vi "Drive Controller.vi"(8 "error out":errorcluster) -> ()   [LabVIEW 2016, in "Drive System.lvlib"]
uses:
  Drive System.lvlib
  Private/DriveCmdList.ctl
  Private/DriveCmd.ctl
  Private/DriveMainType.ctl
  <vilib>/Rock Robotics/WPI/RobotDrive/WPI_RobotDriveDevRef.ctl
  <vilib>/Rock Robotics/WPI/MotorControl/WPI_MotorControlDeviceRef.ctl
  <vilib>/Rock Robotics/WPI/MotorControl/WPI_MotorControlType.ctl
  <vilib>/Rock Robotics/SystemInterfaces/DIO/FPGA_DIOPWMChannel.ctl
  <vilib>/Rock Robotics/WPI/PWM/WPI_PWMDeadband.ctl
  <vilib>/Rock Robotics/WPI/Encoder/WPI_EncoderDevRef.ctl
  <vilib>/Rock Robotics/SystemInterfaces/Encoder/FPGA_EncoderIdx.ctl
  <vilib>/Rock Robotics/SystemInterfaces/Counter/FPGA_CounterCtrSystemIndex.ctl
  <vilib>/Rock Robotics/WPI/Encoder/WPI_EncoderType.ctl
  <vilib>/Rock Robotics/WPI/Gyro/WPI_GyroDevRef.ctl
  <vilib>/Rock Robotics/SystemInterfaces/AI/FPGA_AIChannel.ctl
  <vilib>/Rock Robotics/SystemInterfaces/spilib/spi_bus.ctl
  Private/Varient Cmd Types/Lock Command.ctl
  <vilib>/Rock Robotics/WPI/Solenoid/WPI_SolenoidDevRef.ctl
  <vilib>/Rock Robotics/WPI/Solenoid/WPI_SolenoidChannel.ctl
  Private/Varient Cmd Types/Drive Tank.ctl
  Private/Varient Cmd Types/Drive Arcade.ctl
  Private/Varient Cmd Types/Drive Time.ctl
  Private/Varient Cmd Types/Follow Path.ctl
  Pathfinder/VIs/Segment.ctl
  Private/Raw Data.vi
  <vilib>/Rock Robotics/WPI/Utilities/WPI_GetSetVariantRefNum.vi
  <vilib>/Rock Robotics/Network Tables/NT Write Numeric Array.vi
  <vilib>/Rock Robotics/Network Tables/NT Write String.vi
  Pathfinder/Pathfinder.lvlib
  Private/Drive Refs/Drive Ref Type.ctl
panel:
  out "Locking VI":string
  out "Is Locked?":bool
  out "Active Command:":T1
  out "Visualize":T2(graph)
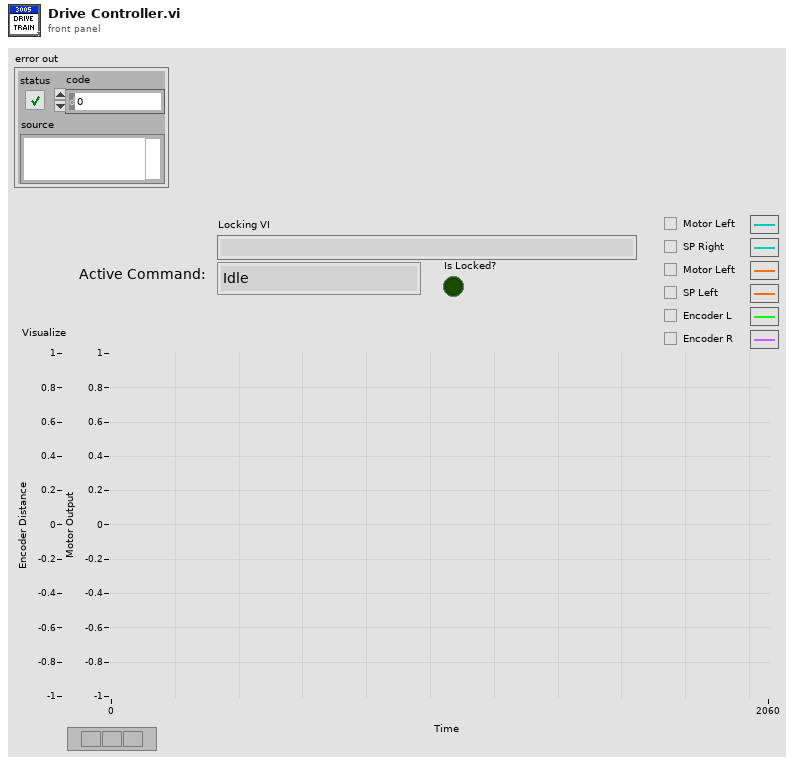
[diagram p1: front panel]
types:
  T1 = typedef "Drive System.lvlib/DriveCmdList.ctl" = enum16{"Idle", "Cleanup", "Drive For Time", "Follow Path Speed Control", "Follow Path", "Drive Tank", "Drive Straight PID", "Drive Angle Mag", "Drive Arcade", "Drive Ref", "Unlock", "Lock"}
  T2 = cluster{"Motor L":dbl, "SP L":dbl, "Motor R":dbl, "SP R":dbl, "Encoder L":dbl, "Encoder R":dbl}
  T3 = typedef "Drive System.lvlib/DriveMainType.ctl" = cluster{"queue":refnum<queue>, "Drivetrain":T4, "Encoder L":T9, "Encoder R":T9, "Gyro":T13, "Lock":T16, "Shifter":T17}
  T4 = typedef "WPI_RobotDriveDevRef.ctl" = cluster{"DevStatus":errorcluster, "Motors[]":T5[], "Square Inputs":bool, "Max Output":dbl}
  T5 = typedef "WPI_MotorControlDeviceRef.ctl" = cluster{"DeviceStatus":errorcluster, "Type":T6, "PWM":cluster{"PWM Channel":T7, "DeadBand":T8}, "CAN":cluster{"Device Number":u8, "SetOutput VI Ref":variant, "GetOutput VI Ref":variant, "Enable VI Ref":variant, "Disable VI Ref":variant, "Data":variant}, "Invert":bool}
  T6 = typedef "WPI_MotorControlType.ctl" = enum16{"PWM", "CAN"}
  T7 = typedef "FPGA_DIOPWMChannel.ctl" = enum8{"PWM 0", "PWM 1", "PWM 2", "PWM 3", "PWM 4", "PWM 5", "PWM 6", "PWM 7", "PWM 8", "PWM 9", "PWM MXP 0", "PWM MXP 1", "PWM MXP 2", "PWM MXP 3", "PWM MXP 4", "PWM MXP 5", "PWM MXP 6", "PWM MXP 7", "PWM MXP 8", "PWM MXP 9", "Invalid"}
  T8 = typedef "WPI_PWMDeadband.ctl" = cluster{"Name":string, "maxPositivePwm":i32, "minPositivePwm":i32, "centerPwm":i32, "maxNegativePwm":i32, "minNegativePwm":i32, "angularRange":u16}
  T9 = typedef "WPI_EncoderDevRef.ctl" = cluster{"DevStatus":errorcluster, "EncoderIndex":T10, "CounterIndex":T11, "DistancePerCount":dbl, "Decoding Type":T12}
  T10 = typedef "FPGA_EncoderIdx.ctl" = enum8{"Enc 0", "Enc 1", "Enc 2", "Enc 3", "Enc 4", "Enc 5", "Enc 6", "Enc 7", "Invalid"}
  T11 = typedef "FPGA_CounterCtrSystemIndex.ctl" = enum8{"Ctr 0", "Ctr 1", "Ctr 2", "Ctr 3", "Ctr 4", "Ctr 5", "Ctr 6", "Ctr 7", "Invalid"}
  T12 = typedef "WPI_EncoderType.ctl" = enum16{"1x", "2x", "4x"}
  T13 = typedef "WPI_GyroDevRef.ctl" = cluster{"DevStatus":errorcluster, "Analog Channel":T14, "Offset":dbl, "Gain (VoltsPerDegree/Second)":dbl, "Gyro Type":enum16{"Analog", "XRS450"}, "Handle":i32, "SPI Bus":T15, "Device Found":bool, "Sample Rate":dbl, "Calibrate On Open":bool}
  T14 = typedef "FPGA_AIChannel.ctl" = enum8{"AI 0", "AI 1", "AI 2", "AI 3", "AI MXP 0", "AI MXP 1", "AI MXP 2", "AI MXP 3", "Invalid"}
  T15 = typedef "spi_bus.ctl" = enum16{"SPI On-Board, CS0", "SPI On-Board, CS1", "SPI On-Board, CS2", "SPI On-Board, CS3", "SPI MXP", "Invalid"}
  T16 = typedef "Drive System.lvlib/Lock Command.ctl" = cluster{"notifier out":refnum<notifier>}
  T17 = typedef "WPI_SolenoidDevRef.ctl" = cluster{"DevStatus":errorcluster, "Pneumatics Control Module":u8, "Forward Solenoid Channel":T18, "Reverse Solenoid Channel":T18}
  T18 = typedef "WPI_SolenoidChannel.ctl" = enum8{"Solenoid 0", "Solenoid 1", "Solenoid 2", "Solenoid 3", "Solenoid 4", "Solenoid 5", "Solenoid 6", "Solenoid 7", "Invalid"}
  T19 = typedef "Drive System.lvlib/DriveCmd.ctl" = cluster{"cmd":T1, "data":variant, "Force? (F)":bool, "Lock":string}
  T20 = typedef "Drive System.lvlib/Drive Tank.ctl" = cluster{"Left":dbl, "Right":dbl}
  T21 = typedef "Drive System.lvlib/Drive Arcade.ctl" = cluster{"X Axis":dbl, "Y Axis":dbl}
  T22 = typedef "Drive System.lvlib/Drive Time.ctl" = cluster{"X Axis":dbl, "Y Axis":dbl, "Time (ms)":u32}
  T23 = typedef "Drive System.lvlib/Follow Path.ctl" = cluster{"Left":T24[], "Right":T24[]}
  T24 = typedef "Pathfinder.lvlib/Segment.ctl" = cluster{"dt":dbl, "x":dbl, "y":dbl, "position":dbl, "velocity":dbl, "acceleration":dbl, "jerk":dbl, "heading":dbl}
  T25 = typedef "Drive System.lvlib/Drive Ref Type.ctl" = refnum<vi>
  T26 = typedef "WPI_DriverStationRobotMode2.ctl" = enum16{"Autonomous Disabled", "Autonomous Enabled", "Teleop Disabled", "Teleop Enabled", "Disconnected", "Finish", "Test Disabled", "Test Enabled", "Emergency Stopped"}
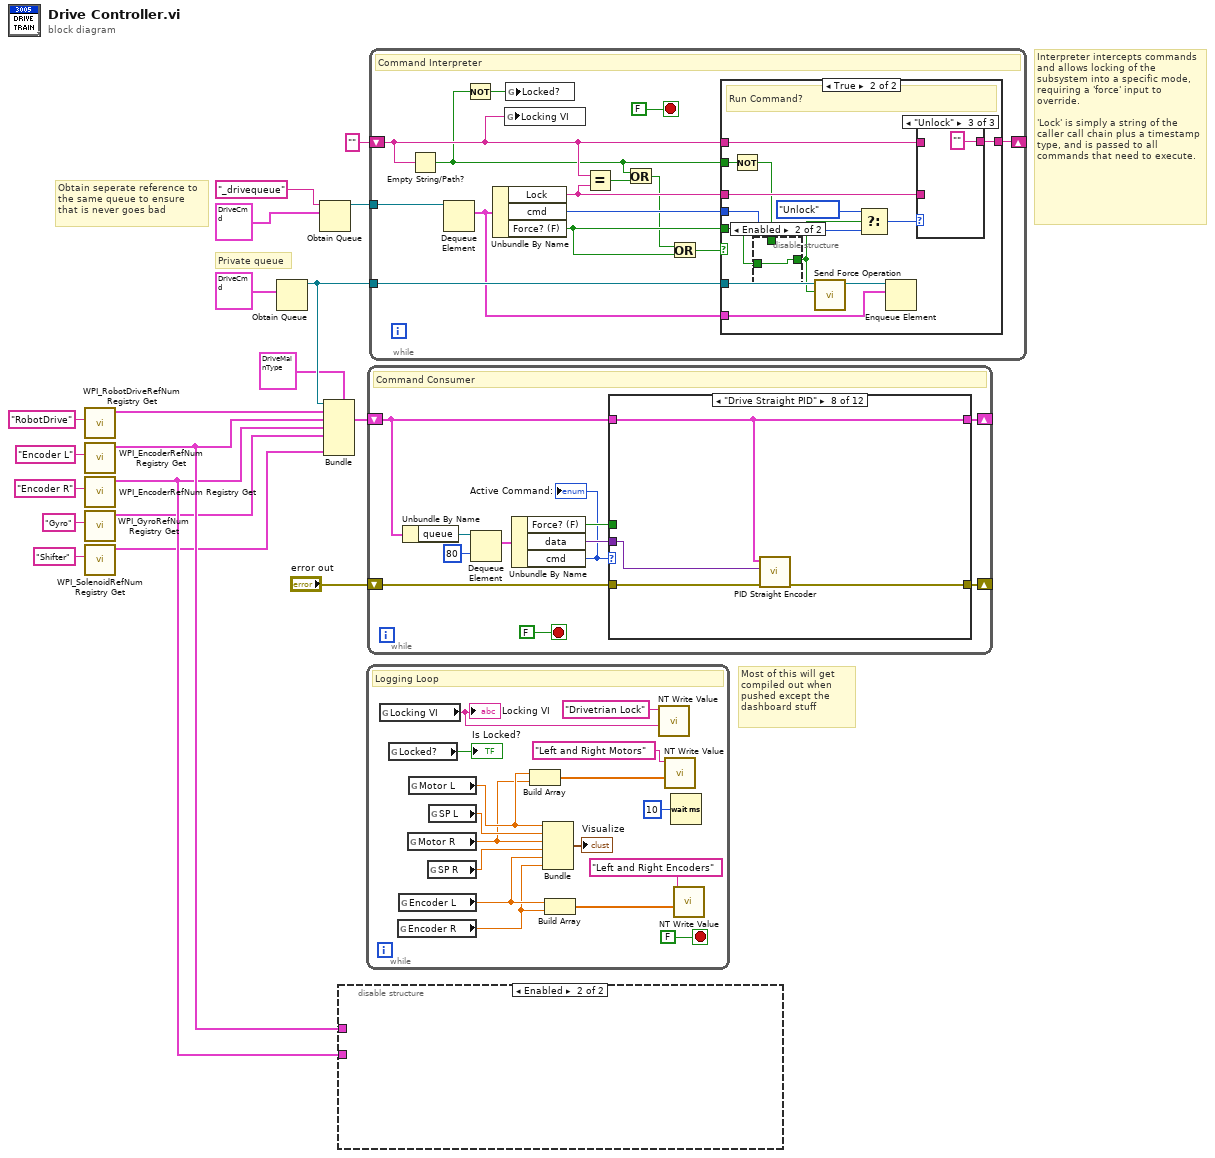
[diagram p0: block diagram]
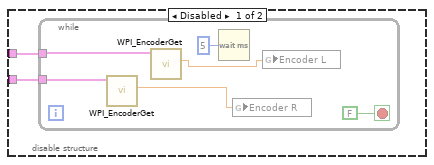
[diagram p2: hidden frame]
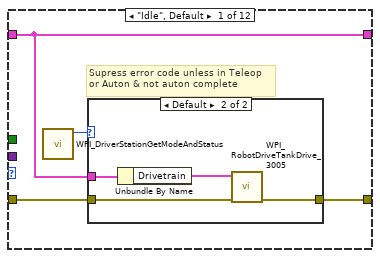
[diagram p3: hidden frame]
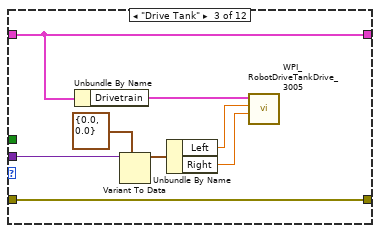
[diagram p6: hidden frame]
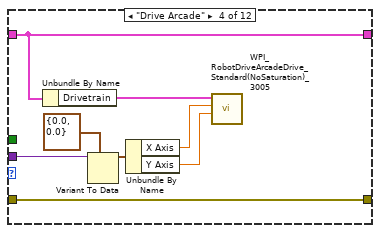
[diagram p7: hidden frame]
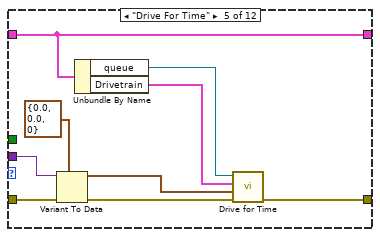
[diagram p8: hidden frame]
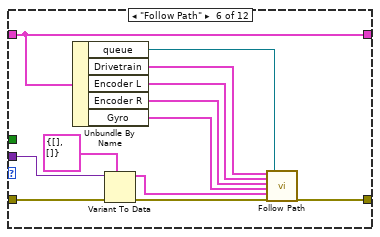
[diagram p9: hidden frame]
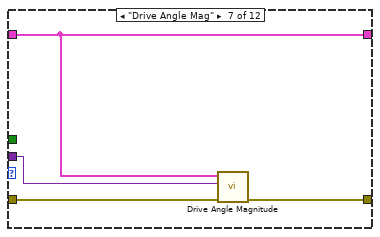
[diagram p10: hidden frame]
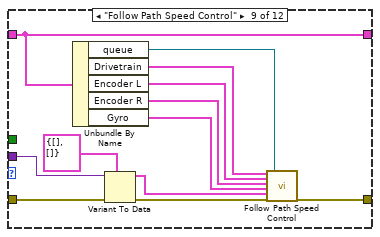
[diagram p11: hidden frame]
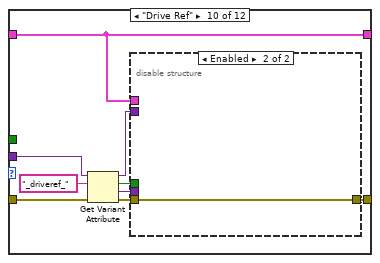
[diagram p12: hidden frame]
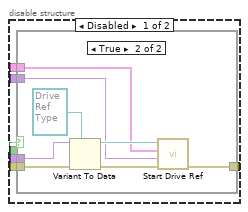
[diagram p13: hidden frame]
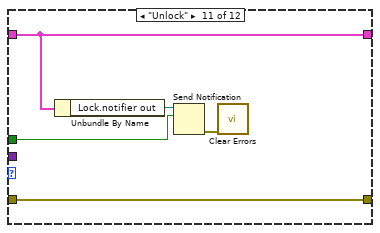
[diagram p15: hidden frame]
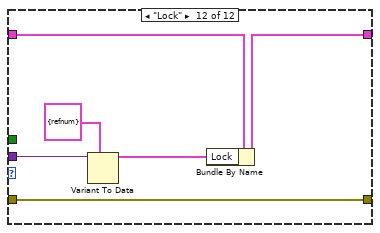
[diagram p16: hidden frame]
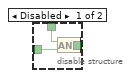
[diagram p18: hidden frame]
diagram:
  # "Most of this will get compiled out when pushed except the dashboard stuff"
  # "Interpreter intercepts commands and allows locking of the subsystem into a specific mode, requiring a 'force' input to override.\n\n'Lock' is simply a string of the caller call chain plus a timestamp type, and is passed to all commands that need to execute."
  # "Private queue"
  # "Obtain seperate reference to\nthe same queue to ensure\nthat is never goes bad"
  n1 = call <vilib>:"WPI_RobotDriveRefNum Registry Get.vi"("refnum name"="RobotDrive") -> ("RobotDriveDevRef"=w4:T4)  [unwired: 9 in, 1 out]
  n2 = call <vilib>:"WPI_EncoderRefNum Registry Get.vi"("refnum name"="Encoder L") -> ("EncoderDevRef"=w7:T9)  [unwired: 9 in, 1 out]
  n3 = call <vilib>:"WPI_EncoderRefNum Registry Get.vi"("refnum name"="Encoder R") -> ("EncoderDevRef"=w6:T9)  [unwired: 9 in, 1 out]
  n4 = call <vilib>:"WPI_GyroRefNum Registry Get.vi"("refnum name"="Gyro") -> ("GyroDevRef"=w5:T13)  [unwired: 9 in, 1 out]
  n5 = call <vilib>:"WPI_SolenoidRefNum Registry Get.vi"("refnum name"="Shifter") -> ("SolenoidDevRef"=w2:T17)  [unwired: 9 in, 1 out]
  n6 = Obtain Queue(element data type=T19 {"cmd"=enum."Cleanup", "data"=variant, "Force? (F)"=FALSE, "Lock"=""} ("Cluster")) -> (queue out=w19:refnum<queue>)  [unwired: 4 in, 2 out]
  n7 = Obtain Queue(name (unnamed)="_drivequeue", element data type=T19 {"cmd"=enum."Cleanup", "data"=variant, "Force? (F)"=FALSE, "Lock"=""}) -> (queue out=w14:refnum<queue>)  [unwired: 3 in, 2 out]
  n8 = Bundle(cluster=T3 {"queue"=refnum, "Drivetrain"={"DevStatus"={"status"=FALSE, "code"=0, "source"=""}, "Motors[]"=[], "Square Inputs"=FALSE, "Max Output"=0.0}, "Encoder L"={"DevStatus"={"status"=FALSE, "code"=0, "source"=""}, "EncoderIndex"=enum."Invalid", "CounterIndex"=enum."Invalid", "DistancePerCount"=1.0, "Decoding Type"=enum."4x"}, "Encoder R"={"DevStatus"={"status"=FALSE, "code"=0, "source"=""}, "EncoderIndex"=enum."Invalid", "CounterIndex"=enum."Invalid", "DistancePerCount"=1.0, "Decoding Type"=enum."4x"}, "Gyro"={"DevStatus"={"status"=FALSE, "code"=0, "source"=""}, "Analog Channel"=enum."Invalid", "Offset"=0.0, "Gain (VoltsPerDegree/Second)"=0.0, "Gyro Type"=enum."Analog", "Handle"=0, "SPI Bus"=enum."Invalid", "Device Found"=FALSE, "Sample Rate"=1.0, "Calibrate On Open"=FALSE}, "Lock"={"notifier out"=refnum}, "Shifter"={"DevStatus"={"status"=FALSE, "code"=0, "source"=""}, "Pneumatics Control Module"=0, "Forward Solenoid Channel"=enum."Invalid", "Reverse Solenoid Channel"=enum."Invalid"}}, "queue"=w19, "Drivetrain"=w4, "Encoder L"=w7, "Encoder R"=w6, "Gyro"=w5, "Shifter"=w2) -> (w18:T3)  [unwired: 1 in]
  n9 = disable-structure shown="Enabled" {
    disable-tunnel: w6 -> [w21 _]
    disable-tunnel: w7 -> [w20 _]
    frame Disabled {
      n10 = while {
        tunnel: w21 -> [w26]
        tunnel: w20 -> [w27]
        stop <- FALSE stop-if-true
        n11 = call <vilib>:"WPI_EncoderGet.vi"("EncoderDevRef"=w26) -> ("Distance"=w22:dbl)  [unwired: 5 in, 5 out]
        n12 = call <vilib>:"WPI_EncoderGet.vi"("EncoderDevRef"=w27) -> ("Distance"=w23:dbl)  [unwired: 5 in, 5 out]
        n13 = Wait (ms)(milliseconds to wait=u32 5) -> ()  [unwired: 1 out]
        n14 = global write "Raw Data.vi" "Encoder R"(w22) -> ()
        n15 = global write "Raw Data.vi" "Encoder L"(w23) -> ()
      }
    }
    frame Enabled {
    }
  }
  n16 = while {
    stop <- FALSE stop-if-true
    # "Logging Loop"
    n17 = global read "Raw Data.vi" "Locking VI"() -> (w28:string)
    "Locking VI" <- w28
    n18 = global read "Raw Data.vi" "Locked?"() -> (→"Is Locked?":bool)
    n19 = global read "Raw Data.vi" "Encoder R"() -> (w31:dbl)
    n20 = global read "Raw Data.vi" "Encoder L"() -> (w32:dbl)
    n21 = global read "Raw Data.vi" "Motor R"() -> (w39:dbl)
    n22 = global read "Raw Data.vi" "Motor L"() -> (w40:dbl)
    n23 = global read "Raw Data.vi" "SP R"() -> (w42:dbl)
    n24 = global read "Raw Data.vi" "SP L"() -> (w43:dbl)
    n25 = Build Array(w40, w39) -> (w38:dbl[])
    n26 = Bundle("Motor L"=w40, "SP L"=w43, "Motor R"=w39, "SP R"=w42, "Encoder L"=w32, "Encoder R"=w31) -> (→"Visualize":T2)  [unwired: 1 in]
    n27 = Build Array(w32, w31) -> (w33:dbl[])
    n28 = call-poly <vilib>:"NT Write Value.vi"("String"=w28, "Name"="Drivetrian Lock") -> ()  [unwired: 9 in, 1 out]
    n29 = call-poly <vilib>:"NT Write Value.vi"("Numeric Array"=w38, "Name"="Left and Right Motors") -> ()  [unwired: 9 in, 1 out]
    n30 = Wait (ms)(milliseconds to wait=u32 10) -> ()  [unwired: 1 out]
    n31 = call-poly <vilib>:"NT Write Value.vi"("Numeric Array"=w33, "Name"="Left and Right Encoders") -> ()  [unwired: 9 in, 1 out]
  }
  n32 = while {
    shift-right: [w50] -> _
    shift-left: w18 -> [w51]
    shift-right: [w48] -> _
    shift-left: "error out" -> [w47]
    stop <- FALSE stop-if-true
    # "Command Consumer"
    n33 = Unbundle By Name(w51) -> ("queue"=w52:refnum<queue>)
    n34 = Dequeue Element(queue=w52, timeout in ms (-1)=80) -> (element=w53:T19)  [unwired: 1 in, 3 out]
    n35 = Unbundle By Name(w53) -> ("Force? (F)"=w45:bool, "data"=w49:variant, "cmd"=w44:T1)
    "Active Command:" <- w44
    n36 = case shown="\"Drive Straight PID\"" w44 {
      tunnel: w51 -> [w56 w64 w73 w81 w84 w100 w106 w107 w120 w123 w151 w157]
      tunnel: [w56 w64 w73 w81 w84 w100 w106 w107 w120 w123 w151 w154] -> w50
      tunnel: w49 -> [_ _ w72 w80 w90 w102 w105 w108 w122 w130 _ w155]
      tunnel: [w57 w65 w68 w74 w86 w97 w103 w109 w117 w126 w152 w158] -> w48
      tunnel: w47 -> [w58 w65 w68 w74 w89 w101 w104 w110 w121 w131 w152 w158]
      tunnel: w45 -> [_ _ _ _ _ _ _ _ _ _ w148 _]
      frame "Idle", Default {
        # "Supress error code unless in Teleop\nor Auton & not auton complete"
        n37 = call <vilib>:"WPI_DriverStationGetModeAndStatus.vi"() -> ("Robot Mode"=w55:T26)  [unwired: 10 in, 1 out]
        n38 = case shown="Default" w55 {
          tunnel: w58 -> [w59 w62]
          tunnel: [w59 w60] -> w57
          tunnel: w56 -> [_ w63]
          frame "Teleop Enabled" {
          }
          frame Default {
            n39 = Unbundle By Name(w63) -> ("Drivetrain"=w61:T4)
            n40 = call "WPI_RobotDriveTankDrive_3005.vi"("error in (no error)"=w62, "RobotDriveDevRef"=w61) -> ("error out"=w60:errorcluster)  [unwired: 8 in, 1 out]
          }
        }
      }
      frame "Cleanup" {
      }
      frame "Drive Tank" {
        n41 = Unbundle By Name(w73) -> ("Drivetrain"=w70:T4)
        n42 = Variant To Data(type=T20 {"Left"=0.0, "Right"=0.0}, Variant=w72) -> (data=w69:T20)  [unwired: 1 in, 1 out]
        n43 = Unbundle By Name(w69) -> ("Left"=w67:dbl, "Right"=w66:dbl)
        n44 = call "WPI_RobotDriveTankDrive_3005.vi"("Right axis value"=w66, "Left axis value"=w67, "RobotDriveDevRef"=w70) -> ()  [unwired: 7 in, 2 out]
      }
      frame "Drive Arcade" {
        n45 = Unbundle By Name(w81) -> ("Drivetrain"=w77:T4)
        n46 = Variant To Data(type=T21 {"X Axis"=0.0, "Y Axis"=0.0}, Variant=w80) -> (data=w79:T21)  [unwired: 1 in, 1 out]
        n47 = Unbundle By Name(w79) -> ("X Axis"=w76:dbl, "Y Axis"=w75:dbl)
        n48 = call "WPI_RobotDriveArcadeDrive_Standard(NoSaturation)_3005.vi"("Y axis value"=w75, "X axis value"=w76, "RobotDriveDevRef"=w77) -> ()  [unwired: 7 in, 2 out]
      }
      frame "Drive For Time" {
        n49 = Variant To Data(error in=w89, type=T22 {"X Axis"=0.0, "Y Axis"=0.0, "Time (ms)"=0} ("Cluster"), Variant=w90) -> (data=w83:T22, error out=w87:errorcluster)
        n50 = Unbundle By Name(w84) -> ("queue"=w85:refnum<queue>, "Drivetrain"=w82:T4)
        n51 = call "Drive for Time.vi"("error in"=w87, "Cluster"=w83, "Drivetrain"=w82, "Queue in"=w85) -> ("error out"=w86:errorcluster)  [unwired: 7 in]
      }
      frame "Follow Path" {
        n52 = Unbundle By Name(w100) -> ("queue"=w94:refnum<queue>, "Drivetrain"=w93:T4, "Encoder L"=w92:T9, "Encoder R"=w91:T9, "Gyro"=w95:T13)
        n53 = Variant To Data(error in=w101, type=T23 {"Left"=[], "Right"=[]}, Variant=w102) -> (data=w96:T23, error out=w98:errorcluster)
        n54 = call "Follow Path.vi"("Drivetrain"=w93, "Encoder L"=w92, "Encoder R"=w91, "Gyro"=w95, "Trajectory"=w96, "error in"=w98, "Queue in"=w94) -> ("error out"=w97:errorcluster)  [unwired: 12 in]
      }
      frame "Drive Angle Mag" {
        n55 = call "Drive Angle Magnitude.vi"("error in"=w104, "data"=w105, "DriveRef"=w106) -> ("error out"=w103:errorcluster)  [unwired: 8 in]
      }
      frame "Drive Straight PID" {
        n56 = call "PID Straight Encoder.vi"("error in"=w110, "data"=w108, "Auton Ref"=w107) -> ("error out"=w109:errorcluster)  [unwired: 8 in]
      }
      frame "Follow Path Speed Control" {
        n57 = Unbundle By Name(w120) -> ("queue"=w114:refnum<queue>, "Drivetrain"=w113:T4, "Encoder L"=w112:T9, "Encoder R"=w111:T9, "Gyro"=w115:T13)
        n58 = Variant To Data(error in=w121, type=T23 {"Left"=[], "Right"=[]}, Variant=w122) -> (data=w116:T23, error out=w118:errorcluster)
        n59 = call "Follow Path Speed Control.vi"("Drivetrain"=w113, "Encoder L"=w112, "Encoder R"=w111, "Gyro"=w115, "Trajectory"=w116, "error in"=w118, "Queue in"=w114) -> ("error out"=w117:errorcluster)  [unwired: 12 in]
      }
      frame "Drive Ref" {
        n60 = Get Variant Attribute(Variant=w130, name="_driveref_", error in=w131) -> (duplicate Variant=w124:variant, found=w125:bool, value=w128:variant, error out=w127:errorcluster)  [unwired: 1 in]
        n61 = disable-structure shown="Enabled" {
          disable-tunnel: w128 -> [w137 _]
          disable-tunnel: w127 -> [w136 w147]
          disable-tunnel: [w135 w147] -> w126
          disable-tunnel: w125 -> [w134 _]
          disable-tunnel: w124 -> [w133 _]
          disable-tunnel: w123 -> [w132 _]
          frame Disabled {
            n62 = case shown="True" w134 {
              tunnel: w137 -> [_ w145]
              tunnel: w136 -> [w138 w144]
              tunnel: [w138 w140] -> w135
              tunnel: w133 -> [_ w141]
              tunnel: w132 -> [_ w142]
              frame False {
              }
              frame True {
                n63 = Variant To Data(error in=w144, type=T25 refnum ("Drive Ref"), Variant=w145) -> (data=w143:T25, error out=w139:errorcluster)
                n64 = call "Start Drive Ref.vi"("error in"=w139, "Variant"=w141, "cluster"=w142, "VI in"=w143) -> ("error out"=w140:errorcluster)  [unwired: 7 in]
              }
            }
          }
          frame Enabled {
          }
        }
      }
      frame "Unlock" {
        n65 = Unbundle By Name(w151) -> ("Lock.notifier out"=w150:refnum<notifier>)
        n66 = Send Notification(notification=w148, notifier=w150) -> (error out=w149:errorcluster)  [unwired: 1 in, 1 out]
        n67 = call <vilib>:"Clear Errors.vi"("error in (no error)"=w149) -> ()  [unwired: 5 in, 2 out]
      }
      frame "Lock" {
        n68 = Variant To Data(type=T16 {"notifier out"=refnum} ("Cluster"), Variant=w155) -> (data=w153:T16)  [unwired: 1 in, 1 out]
        n69 = Bundle By Name(cluster=w157, "Lock"=w153) -> (w154:T3)
      }
    }
  }
  n70 = while {
    tunnel: w14 -> [w170]
    tunnel: w19 -> [w172]
    shift-right: [w169] -> _
    shift-left: "" -> [w161]
    stop <- FALSE stop-if-true
    # "Command Interpreter"
    n71 = Empty String/Path?(string/path=w161) -> (empty?=w160:bool)
    n72 = Dequeue Element(queue=w170) -> (element=w171:T19)  [unwired: 2 in, 3 out]
    n73 = Not(x=w160) -> (.not. x?=w159:bool)
    n74 = Unbundle By Name(w171) -> ("Lock"=w164:string, "cmd"=w168:T1, "Force? (F)"=w166:bool)
    n75 = global write "Raw Data.vi" "Locking VI"(w161) -> ()
    n76 = global write "Raw Data.vi" "Locked?"(w159) -> ()
    n77 = Equal?(x=w161, y=w164) -> (x = y?=w163:bool)
    n78 = Or(x=w160, y=w163) -> (x .or. y?=w162:bool)
    n79 = Or(x=w162, y=w166) -> (x .or. y?=w167:bool)
    n80 = case shown="True" w167 {
      tunnel: w172 -> [_ w186]
      tunnel: w171 -> [_ w184]
      tunnel: w160 -> [_ w180]
      tunnel: [w173 w179] -> w169
      tunnel: w161 -> [w173 w178]
      tunnel: w166 -> [_ w177]
      tunnel: w168 -> [_ w176]
      tunnel: w164 -> [_ w175]
      frame False {
        # "Locked"
      }
      frame True {
        # "Run Command?"
        n81 = Not(x=w180) -> (.not. x?=w174:bool)
        n82 = disable-structure shown="Enabled" {
          disable-tunnel: [w189 w190] -> w182
          disable-tunnel: w177 -> [w188 w190]
          disable-tunnel: w174 -> [w187 _]
          frame Disabled {
            n83 = And(x=w187, y=w188) -> (x .and. y?=w189:bool)
          }
          frame Enabled {
          }
        }
        n84 = call "Send Force Operation.vi"("Force?"=w182, "queue in"=w186) -> ("queue out"=w185:refnum<queue>)  [unwired: 8 in, 1 out]
        n85 = Select(t=DriveCmdList."Unlock", s=w182, f=w176) -> (s? t:f=w183:T1)
        n86 = Enqueue Element(queue=w185, element=w184) -> ()  [unwired: 2 in, 3 out]
        n87 = case shown="\"Unlock\"" w183 {
          tunnel: w178 -> [w191 _ _]
          tunnel: [w191 w192 ""] -> w179
          tunnel: w175 -> [_ w192 _]
          frame Default {
          }
          frame "Lock" {
          }
          frame "Unlock" {
          }
        }
      }
    }
  }
